vi "Break Container Lease.vi"(8 "error in (no error)":errorcluster, 9 "Break period in seconds (-1: none)":i32=-1, 10 "Container":string, 11 "Azure Session in":refnum<class "Session.lvclass">) -> (0 "error out":errorcluster, 3 "Azure Session out":refnum<class "Session.lvclass">)   [LabVIEW 2015, in "NI_Azure_Blob.lvlib"]
doc: "End the lease on a container but ensure that another client cannot acquire a new lease until the current lease period has expired."
uses:
  NI_Azure_Blob.lvlib
  Core/Session/Session.lvclass
  Core/Name Value Pair.ctl
  Lease Action.ctl
  Core/Session/Session.lvclass/Session.ctl
  Core/Session/Write Request Headers.vi
  Core/Session/Write Request Parameters.vi
  Core/Session/Write HTTP Verb.vi
  Core/Session/Write URL Suffix.vi
  Strings Global.vi
  Core/NI_Azure_Core.lvlib
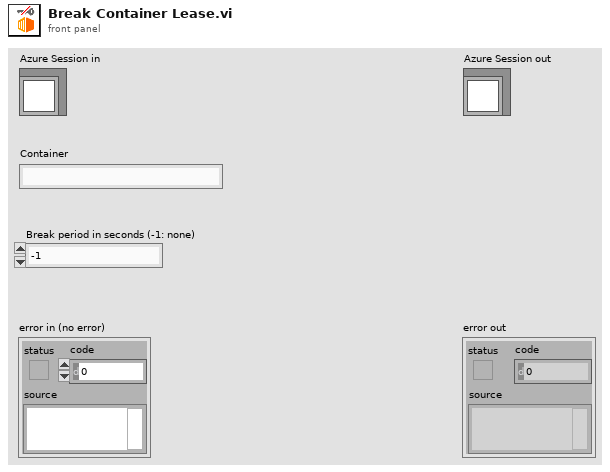
[diagram p1: front panel]
types:
  T1 = typedef "NI_Azure_Blob.lvlib/Lease Action.ctl" = enum16{"acquire", "renew", "change", "release", "break"}
  T2 = typedef "NI_Azure_Core.lvlib/Name Value Pair.ctl" = cluster{"name":string, "value":string}
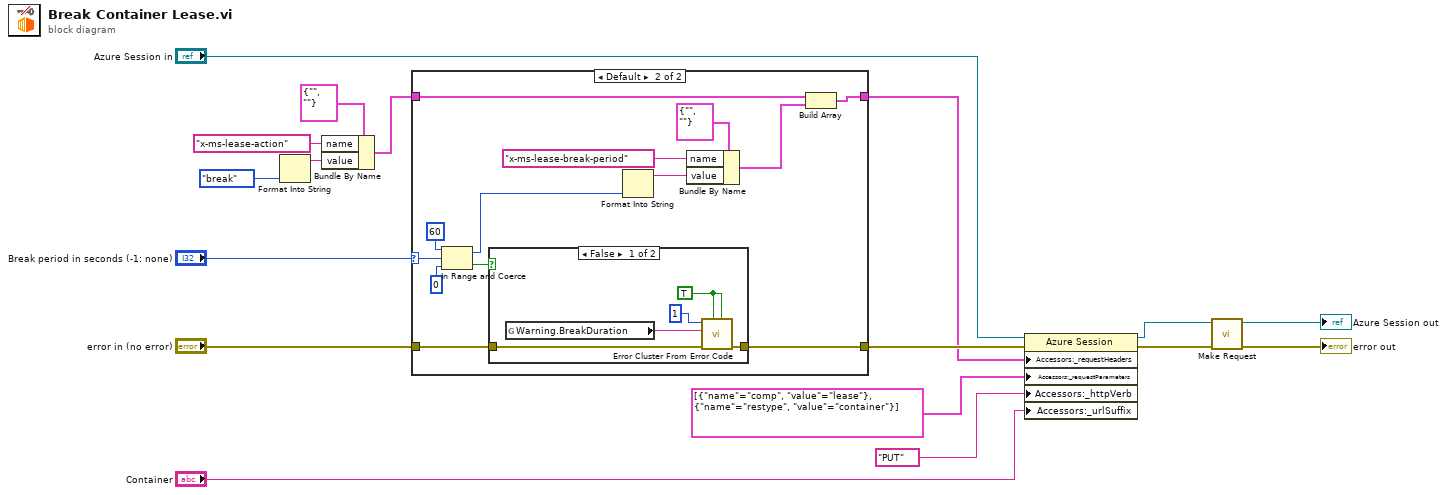
[diagram p0: block diagram]
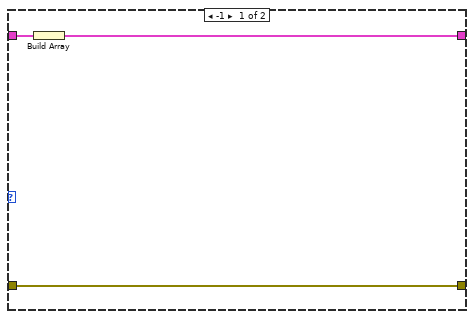
[diagram p2: hidden frame]
diagram:
  n1 = Format Into String(Lease_Action."break" ("Lease action")) -> (resulting string=w12:string)  [unwired: 3 in, 1 out]
  n2 = Bundle By Name(cluster=T2 {"name"="", "value"=""} ("Cluster"), "name"="x-ms-lease-action" ("header"), "value"=w12) -> (w8:T2)
  n3 = case shown="Default" "Break period in seconds (-1: none)" {
    selector: "Break period in seconds (-1: none)" -> [_ w28]
    tunnel: "error in (no error)" -> [w20 w30]
    tunnel: [w20 w29] -> w9
    tunnel: w8 -> [w19 w23]
    tunnel: [w18 w21] -> w4
    frame -1 {
      n4 = Build Array(w19) -> (w18:T2[])
    }
    frame Default {
      n5 = In Range and Coerce(upper limit=60, x=w28, lower limit=0) -> (coerced(x)=w27:i32, In Range?=w24:bool)
      n6 = case shown="False" w24 {
        tunnel: w30 -> [w37 w39]
        tunnel: [w36 w39] -> w29
        frame False {
          w38 = TRUE ("show call chain? (False)")
          n7 = global read "Strings Global.vi" "Warning.BreakDuration"() -> (w34:string)
          n8 = call <vilib>:"Error Cluster From Error Code.vi"("is warning? (False)"=w38, "show call chain? (False)"=w38, "error in (no error)"=w37, "error message (\"\")"=w34, "error code (0)"=1) -> ("error out"=w36:errorcluster)  [unwired: 4 in]
        }
        frame True {
        }
      }
      n9 = Format Into String(w27) -> (resulting string=w32:string)  [unwired: 3 in, 1 out]
      n10 = Bundle By Name(cluster=T2 {"name"="", "value"=""} ("Cluster"), "name"="x-ms-lease-break-period" ("header"), "value"=w32) -> (w22:T2)
      n11 = Build Array(w23, w22) -> (w21:T2[])
    }
  }
  n12 = property class="Azure Session"(reference="Azure Session in", error in=w9, "Accessors:_requestHeaders"=w4, "Accessors:_requestParameters"=T2[] [{"name"="comp", "value"="lease"}, {"name"="restype", "value"="container"}] ("request parameters"), "Accessors:_httpVerb"="PUT" ("HTTP-Verb"), "Accessors:_urlSuffix"="Container") -> (reference out=w5:refnum<class "Session.lvclass">, error out=w7:errorcluster)
  n13 = call "Make Request.vi"("error in (no error)"=w7, "Session in"=w5) -> ("error out"=→"error out":errorcluster, "Session out"=→"Azure Session out":refnum<class "Session.lvclass">)  [unwired: 7 in, 1 out]
